vi "Day11-2.vi"() -> ()   [LabVIEW 2021]
panel:
  out "Step":i32
  out "Array":i32[][](array[numeric])
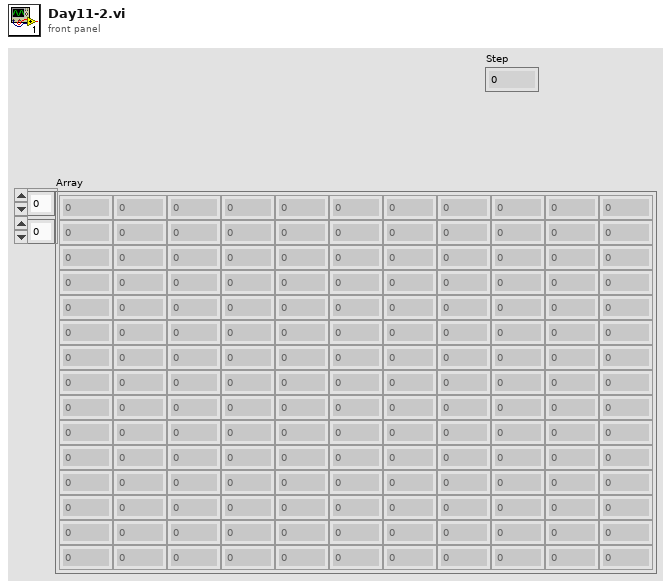
[diagram p1: front panel]
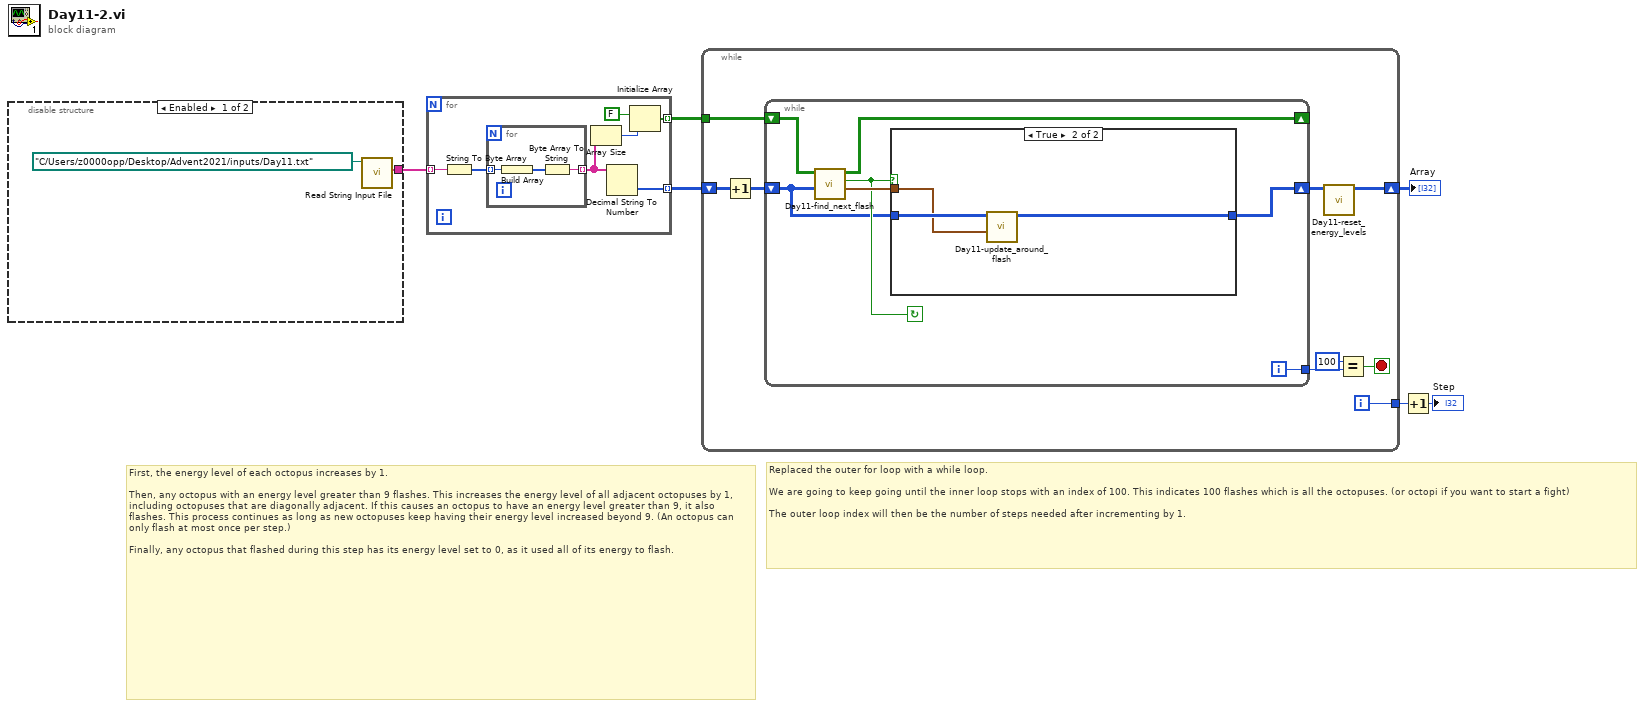
[diagram p0: block diagram]
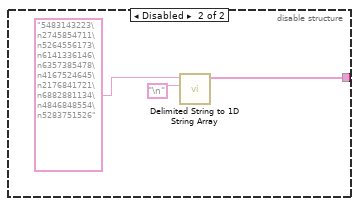
[diagram p3: hidden frame]
diagram:
  # "Replaced the outer for loop with a while loop.\n\nWe are going to keep going until the inner loop stops with an index of 100. This indicates 100 flashes which is all the octopuses. (or octopi if you want to start a fight)\n\nThe outer loop index will then be the number of steps needed after incrementing by 1."
  # "First, the energy level of each octopus increases by 1.\n\nThen, any octopus with an energy level greater than 9 flashes. This increases the energy level of all adjacent octopuses by 1, including octopuses that are diagonally adjacent. If this causes an octopus to have an energy level greater than 9, it also flashes. This process continues as long as new octopuses keep having their energy level increased beyond 9. (An octopus can only flash at most once per step.)\n\nFinally, any octopus that flashed during this step has its energy level set to 0, as it used all of its energy to flash."
  n1 = disable-structure shown="Enabled" {
    disable-tunnel: [w7 w9] -> w6
    frame Enabled {
      n2 = call "Read String Input File.vi"("file path (dialog if empty)"=path "C:/Users/z0000opp/Desktop/Advent2021/inputs/Day11.txt") -> ("input values"=w7:string[])  [unwired: 10 in]
    }
    frame Disabled {
      n3 = call <vilib>:"Delimited String to 1D String Array.vi"("delimiter"="\n", "delimited string"="5483143223\n2745854711\n5264556173\n6141336146\n6357385478\n4167524645\n2176841721\n6882881134\n4846848554\n5283751526") -> ("string array"=w9:string[])  [unwired: 9 in]
    }
  }
  n4 = for {
    tunnel: w6 -> [w18] mode=indexing
    tunnel: [w16] -> w5 mode=indexing
    tunnel: [w12] -> w3 mode=indexing
    n5 = String To Byte Array(string=w18) -> (unsigned byte array=w17:u8[])
    n6 = for {
      tunnel: w17 -> [w21] mode=indexing
      tunnel: [w19] -> w14 mode=indexing
      n7 = Build Array(w21) -> (w20:u8[])
      n8 = Byte Array To String(unsigned byte array=w20) -> (string=w19:string)
    }
    n9 = Array Size(array=w14) -> (size(s)=w13:i32)
    n10 = Decimal String To Number(string=w14) -> (number=w16:i32[])  [unwired: 2 in, 1 out]
    n11 = Initialize Array(FALSE, w13) -> (w12:bool[])
  }
  n12 = while {
    shift-right: [w26] -> w4
    shift-left: w5 -> [w30]
    tunnel: w3 -> [w28]
    tunnel: [w22] -> w2
    i -> [w22]
    stop <- w23 stop-if-true
    n13 = Increment(x=w30) -> (x+1=w29:i32[][])
    n14 = while {
      shift-right: [w32] -> w27
      shift-left: w29 -> [w33]
      shift-right: [w36] -> _
      shift-left: w28 -> [w37]
      tunnel: [w31] -> w25
      i -> [w31]
      stop <- w34 continue-if-true
      n15 = call "Day11-find_next_flash.vi"("Energy Levels"=w33, "Flashed"=w37) -> ("Flash Location"=w35:cluster{i32, i32}, "New Flash?"=w34:bool, "Flashed out"=w36:bool[][])  [unwired: 7 in]
      n16 = case shown="True" w34 {
        tunnel: w35 -> [_ w40]
        tunnel: w33 -> [w38 w41]
        tunnel: [w38 w39] -> w32
        frame False {
        }
        frame True {
          n17 = call "Day11-update_around_flash.vi"("Flash Location"=w40, "Energy Levels"=w41) -> ("Energy Levels out"=w39:i32[][])  [unwired: 9 in]
        }
      }
    }
    n18 = call "Day11-reset_energy_levels.vi"("Energy Levels"=w27) -> ("Energy Levels out"=w26:i32[][])  [unwired: 10 in]
    n19 = Equal?(x=100, y=w25) -> (x = y?=w23:bool)
  }
  "Array" <- w4
  n20 = Increment(x=w2) -> (x+1=→"Step":i32)
